vi "DqmhModuleDiagramGraph_Create.vi"(0 "reference in":refnum<class "DqmhModuleDiagramGraph.lvclass">, 5 "error in (no error)":errorcluster) -> (14 "reference out":refnum<class "DqmhModuleDiagramGraph.lvclass">, 19 "error out":errorcluster)   [LabVIEW 2016, in "DqmhModuleDiagramGraph.lvclass"]
doc: "Creates and initializes a new ClassDiagramGraph object.\n\nThis object should be destroyed using a ClassDiagramGraph destructor VI or a virtual base class destructor VI.\n\n[GOOP 2.1]"
uses:
  <resource>/Framework/Providers/Open_GDS/UML/DqmhModuleDiagramGraph_class/DqmhModuleDiagramGraph.lvclass
  C:/Program Files (x86)/National Instruments/LabVIEW 2016/resource/Framework/Providers/Open_GDS/UML/Graph_class/Graph.lvclass
  <resource>/Framework/Providers/Open_GDS/UML/Graph_class/Graph.lvclass
  <resource>/Framework/Providers/Open_GDS/UML/DQMH_API_class/DQMH_API.lvclass
panel:
  # "The input reference should only\nbe wired when this method is called\nby a sub class constructor."
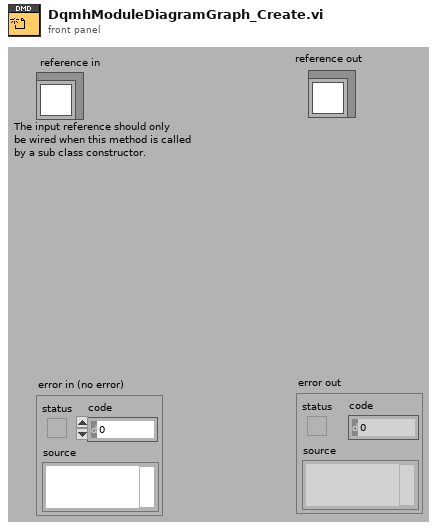
[diagram p1: front panel]
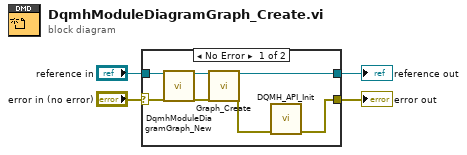
[diagram p0: block diagram]
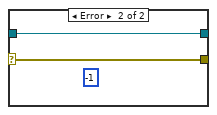
[diagram p2: hidden frame]
diagram:
  n1 = case shown="No Error" "error in (no error)" {
    selector: "error in (no error)" -> [w11 w13]
    tunnel: [w8 w12] -> w4
    tunnel: [w5 w13] -> w3
    tunnel: "reference in" -> [w10 w12]
    frame No Error {
      n2 = call <resource>:"DqmhModuleDiagramGraph_New.vi"("reference in"=w10, "error in (no error)"=w11) -> ("reference out"=w9:refnum<class "DqmhModuleDiagramGraph.lvclass">, "error out"=w7:errorcluster)  [unwired: 2 in, 14 out]
      n3 = call <resource>:"Graph_Create.vi"("reference"=w9, "error in (no error)"=w7) -> ("reference out"=w8:refnum<class "DqmhModuleDiagramGraph.lvclass">, "error out"=w6:errorcluster)  [unwired: 1 in, 15 out]
      n4 = call <resource>:"DQMH_API_Init.vi"("error in (no error)"=w6) -> ("error out"=w5:errorcluster)  [unwired: 13 in, 1 out]
    }
    frame Error {
      (unwired) -1 ("Nr of open handles")
    }
  }
  "error out" <- w3
  "reference out" <- w4
